vi "Z900_navX_SERIAL_DecodePacket.vi"(8 "error in (no error)":errorcluster, 10 "Data":u8[](array[numeric]), 11 "Packet":string) -> (0 "error out":errorcluster, 2 "Data":u8[](array[numeric]), 3 "Packet":string)   [LabVIEW 2015, in "navX Library v2.lvlib"]
uses:
  navX Library v2.lvlib
  TypeDefs/Z900_navX_DeviceRegisters.ctl
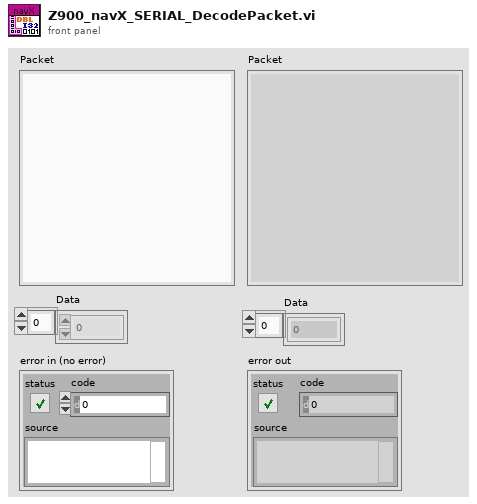
[diagram p1: front panel]
types:
  T1 = typedef "navX Library v2.lvlib/Z900_navX_DeviceRegisters.ctl" = u8
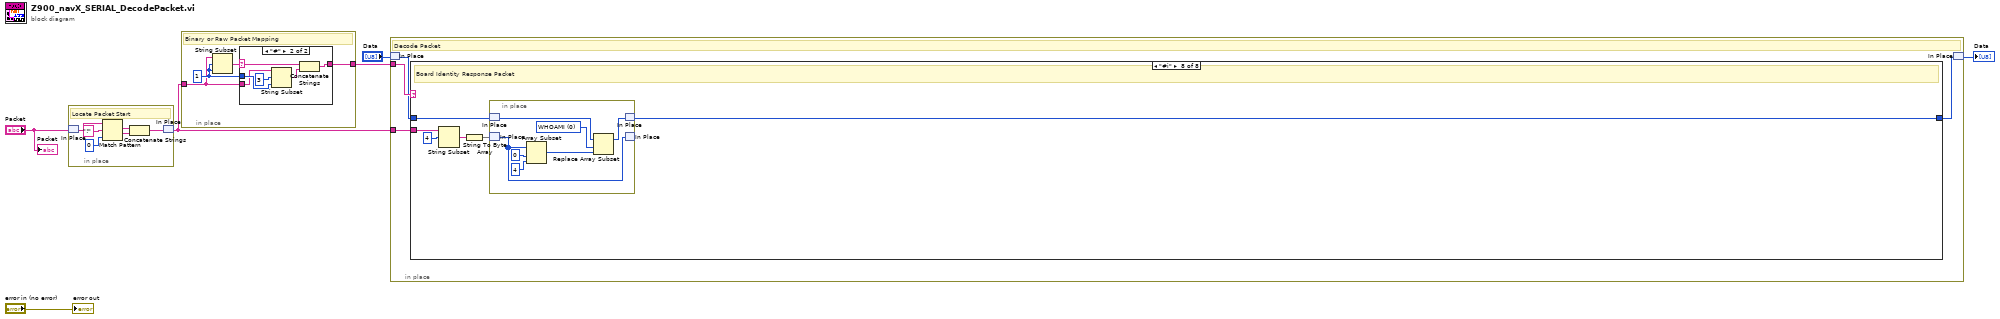
[diagram p0: block diagram]
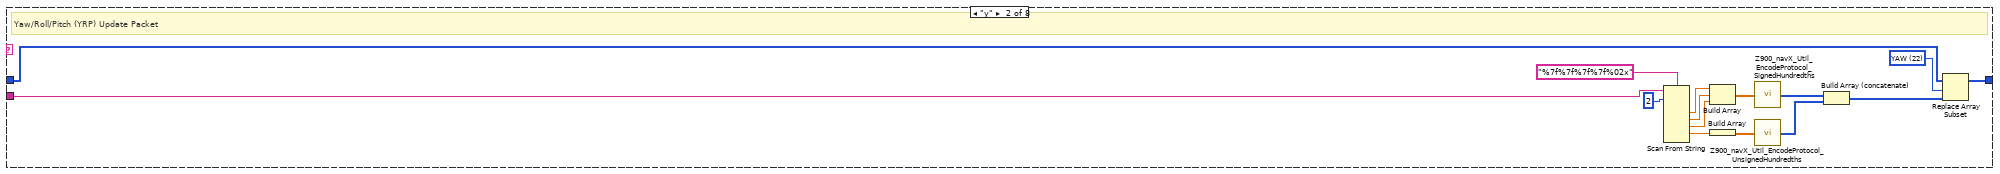
[diagram p3: hidden frame]
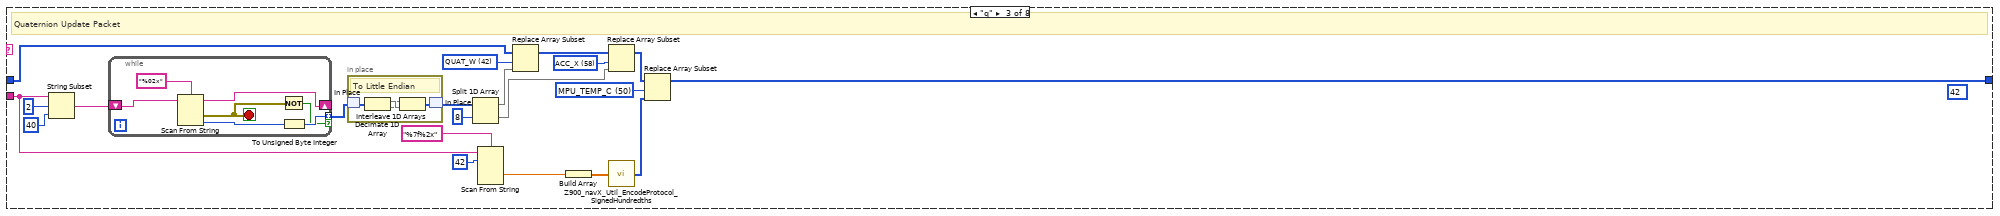
[diagram p4: hidden frame]
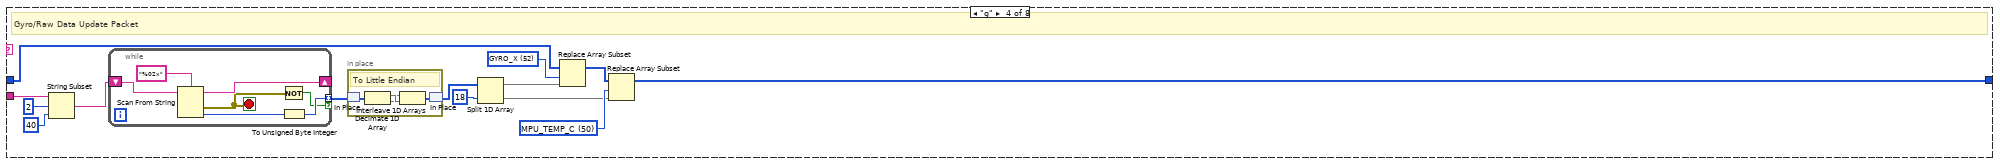
[diagram p5: hidden frame]
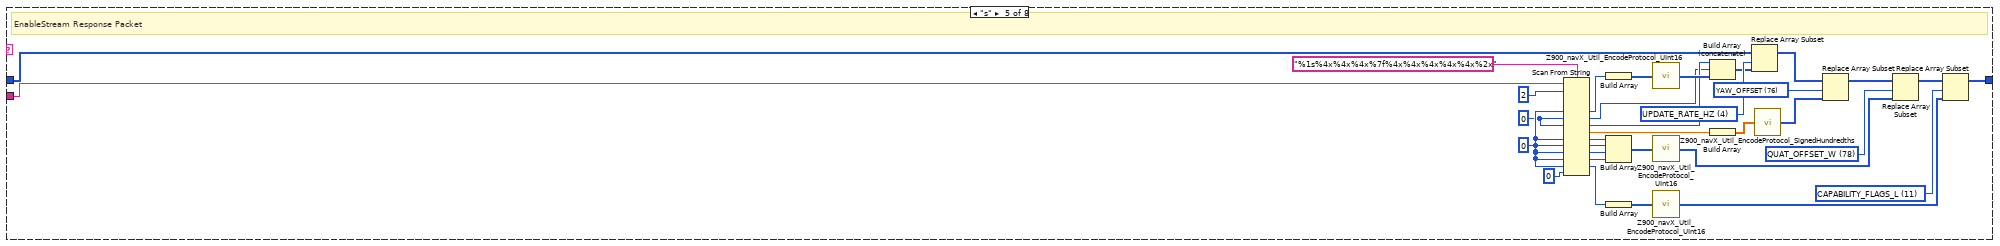
[diagram p6: hidden frame]
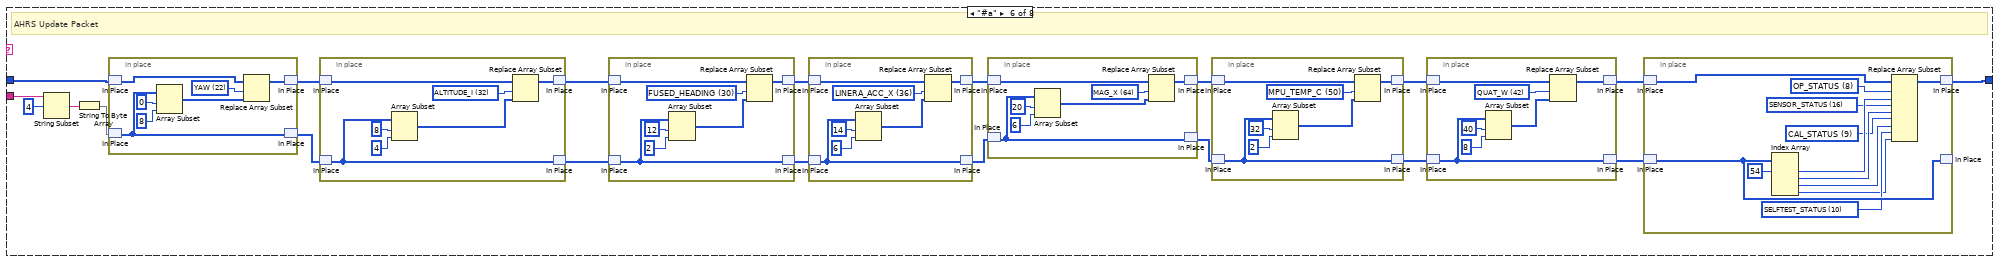
[diagram p7: hidden frame]
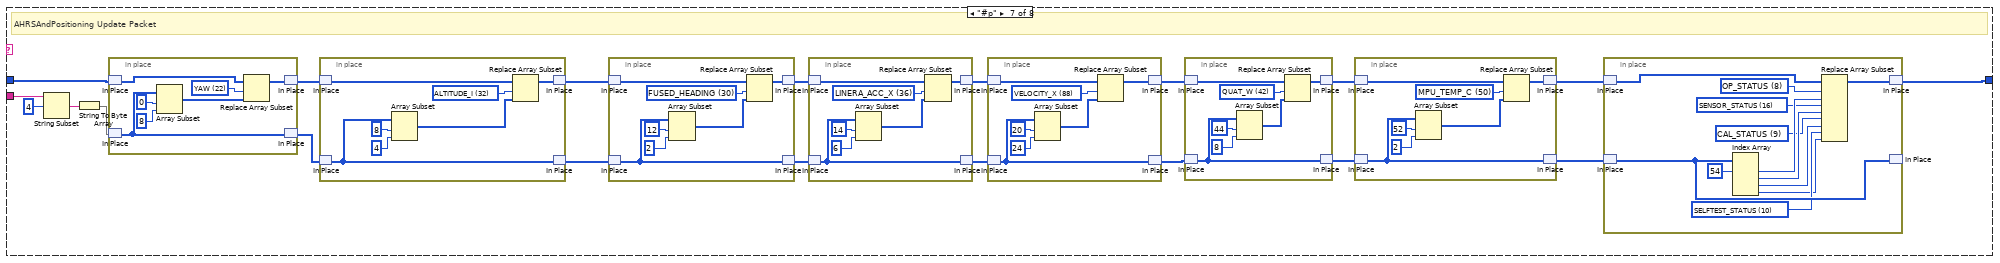
[diagram p8: hidden frame]
diagram:
  n1 = in-place {
    # "Locate Packet Start"
    n2 = in-place-match #1("Packet") -> (w8:string)
    n3 = Match Pattern(string=w8, regular expression="!" ("Packet Start Char"), offset (0)=0 ("offset past match")) -> (match substring=w11:string, after substring=w10:string)  [unwired: 2 out]
    n4 = Concatenate Strings(w11, w10) -> (w7:string)
    n5 = in-place-match #1(w7) -> (w2:string)
  }
  n6 = in-place {
    in-place-border: w2 -> [w14]
    in-place-border: [w16] -> w3
    w15 = 1 ("length (rest)")
    # "Binary or Raw Packet Mapping"
    n7 = String Subset(string=w14, offset (0)=w15, length (rest)=w15) -> (substring=w13:string)
    n8 = case shown="\"#\"" w13 {
      selector: w13 -> [w17 w18]
      tunnel: [w17 w19] -> w16
      tunnel: w15 -> [_ w22]
      tunnel: w14 -> [_ w21]
      frame Default {
      }
      frame "#" {
        n9 = String Subset(string=w21, offset (0)=3, length (rest)=w22) -> (substring=w20:string)
        n10 = Concatenate Strings(w18, w20) -> (w19:string)
      }
    }
  }
  n11 = in-place {
    in-place-border: w3 -> [w27]
    in-place-border: w2 -> [w25]
    # "Decode Packet"
    n12 = in-place-match #2("Data") -> (w26:u8[])
    n13 = case shown="\"#i\"" w27 {
      tunnel: w26 -> [w28 w34 w48 w85 w122 w150 w230 w297]
      tunnel: [w28 w29 w54 w78 w111 w134 w215 w296] -> w24
      tunnel: w25 -> [_ w41 w59 w87 w128 w153 w231 w299]
      frame Default {
        # "We should not care about decoding this packet type."
        # "Unknown Packet"
      }
      frame "y" {
        w30 = T1 22 items=["WHOAMI"=0, "HW_REV"=1, "FW_VER_MAJOR"=2, "FW_VER_MINOR"=3, "UPDATE_RATE_HZ"=4, "ACCEL_FSR_G"=5, "GYRO_FSR_DPS"=6, "OP_STATUS"=8, "CAL_STATUS"=9, "SELFTEST_STATUS"=10, "CAPABILITY_FLAGS_L"=11, "CAPABILITY_FLAGS_H"=12, "SENSOR_STATUS"=16, "TIMESTAMP"=18, "YAW"=22, "ROLL"=24, "PITCH"=26, "HEADING"=28, "FUSED_HEADING"=30, "ALTITUDE_I"=32, "ALTITUDE_D"=34, "LINERA_ACC_X"=36, "LINERA_ACC_Y"=38, "LINERA_ACC_Z"=40, "QUAT_W"=42, "QUAT_X"=44, "QUAT_Y"=46, "QUAT_Z"=48, "MPU_TEMP_C"=50, "GYRO_X"=52, "GYRO_Y"=54, "GYRO_Z"=56, "ACC_X"=58, "ACC_Y"=60, "ACC_Z"=62, "MAG_X"=64, "MAG_Y"=66, "MAG_Z"=68, "PRESSURE_I"=70, "PRESSURE_D"=72, "PRESSURE_TEMP"=74, "YAW_OFFSET"=76, "QUAT_OFFSET_W"=78, "QUAT_OFFSET_X"=80, "QUAT_OFFSET_Y"=82, "QUAT_OFFSET_Z"=84, "INTEGRATION_CONTROL"=86, "VELOCITY_X"=88, "VELOCITY_Y"=92, "VELOCITY_Z"=96, "DISPLACMENT_X"=100, "DISPLACMENT_Y"=104, "DISPLACEMENT_Z"=108] ("Device Register")
        # "Yaw/Roll/Pitch (YRP) Update Packet"
        n14 = Scan From String(format string="%7f%7f%7f%7f%02x", input string=w41, initial scan location=2 ("offset (0)")) -> (output 1=w40:dbl, output 2=w39:dbl, output 3=w38:dbl, output 4=w36:dbl)  [unwired: 7 in, 3 out]
        n15 = Build Array(w40, w39, w38) -> (w37:dbl[])
        n16 = Build Array(w36) -> (w35:dbl[])
        n17 = call "Z900_navX_Util_EncodeProtocol_SignedHundredths.vi"("Signed Hundredths (0.00)"=w37) -> ("Little Endian"=w33:u8[])
        n18 = call "Z900_navX_Util_EncodeProtocol_UnsignedHundredths.vi"("Unsigned Hundredths (0.00)"=w35) -> ("Little Endian"=w32:u8[])
        n19 = Build Array (concatenate)(w33, w32) -> (w31:u8[])
        n20 = Replace Array Subset(array=w34, new element=w31, index=w30) -> (w29:u8[])
      }
      frame "q" {
        w44 = T1 42 items=["WHOAMI"=0, "HW_REV"=1, "FW_VER_MAJOR"=2, "FW_VER_MINOR"=3, "UPDATE_RATE_HZ"=4, "ACCEL_FSR_G"=5, "GYRO_FSR_DPS"=6, "OP_STATUS"=8, "CAL_STATUS"=9, "SELFTEST_STATUS"=10, "CAPABILITY_FLAGS_L"=11, "CAPABILITY_FLAGS_H"=12, "SENSOR_STATUS"=16, "TIMESTAMP"=18, "YAW"=22, "ROLL"=24, "PITCH"=26, "HEADING"=28, "FUSED_HEADING"=30, "ALTITUDE_I"=32, "ALTITUDE_D"=34, "LINERA_ACC_X"=36, "LINERA_ACC_Y"=38, "LINERA_ACC_Z"=40, "QUAT_W"=42, "QUAT_X"=44, "QUAT_Y"=46, "QUAT_Z"=48, "MPU_TEMP_C"=50, "GYRO_X"=52, "GYRO_Y"=54, "GYRO_Z"=56, "ACC_X"=58, "ACC_Y"=60, "ACC_Z"=62, "MAG_X"=64, "MAG_Y"=66, "MAG_Z"=68, "PRESSURE_I"=70, "PRESSURE_D"=72, "PRESSURE_TEMP"=74, "YAW_OFFSET"=76, "QUAT_OFFSET_W"=78, "QUAT_OFFSET_X"=80, "QUAT_OFFSET_Y"=82, "QUAT_OFFSET_Z"=84, "INTEGRATION_CONTROL"=86, "VELOCITY_X"=88, "VELOCITY_Y"=92, "VELOCITY_Z"=96, "DISPLACMENT_X"=100, "DISPLACMENT_Y"=104, "DISPLACEMENT_Z"=108] ("Device Register")
        w51 = T1 58 items=["WHOAMI"=0, "HW_REV"=1, "FW_VER_MAJOR"=2, "FW_VER_MINOR"=3, "UPDATE_RATE_HZ"=4, "ACCEL_FSR_G"=5, "GYRO_FSR_DPS"=6, "OP_STATUS"=8, "CAL_STATUS"=9, "SELFTEST_STATUS"=10, "CAPABILITY_FLAGS_L"=11, "CAPABILITY_FLAGS_H"=12, "SENSOR_STATUS"=16, "TIMESTAMP"=18, "YAW"=22, "ROLL"=24, "PITCH"=26, "HEADING"=28, "FUSED_HEADING"=30, "ALTITUDE_I"=32, "ALTITUDE_D"=34, "LINERA_ACC_X"=36, "LINERA_ACC_Y"=38, "LINERA_ACC_Z"=40, "QUAT_W"=42, "QUAT_X"=44, "QUAT_Y"=46, "QUAT_Z"=48, "MPU_TEMP_C"=50, "GYRO_X"=52, "GYRO_Y"=54, "GYRO_Z"=56, "ACC_X"=58, "ACC_Y"=60, "ACC_Z"=62, "MAG_X"=64, "MAG_Y"=66, "MAG_Z"=68, "PRESSURE_I"=70, "PRESSURE_D"=72, "PRESSURE_TEMP"=74, "YAW_OFFSET"=76, "QUAT_OFFSET_W"=78, "QUAT_OFFSET_X"=80, "QUAT_OFFSET_Y"=82, "QUAT_OFFSET_Z"=84, "INTEGRATION_CONTROL"=86, "VELOCITY_X"=88, "VELOCITY_Y"=92, "VELOCITY_Z"=96, "DISPLACMENT_X"=100, "DISPLACMENT_Y"=104, "DISPLACEMENT_Z"=108] ("Device Register")
        (unwired) T1 42 items=["WHOAMI"=0, "HW_REV"=1, "FW_VER_MAJOR"=2, "FW_VER_MINOR"=3, "UPDATE_RATE_HZ"=4, "ACCEL_FSR_G"=5, "GYRO_FSR_DPS"=6, "OP_STATUS"=8, "CAL_STATUS"=9, "SELFTEST_STATUS"=10, "CAPABILITY_FLAGS_L"=11, "CAPABILITY_FLAGS_H"=12, "SENSOR_STATUS"=16, "TIMESTAMP"=18, "YAW"=22, "ROLL"=24, "PITCH"=26, "HEADING"=28, "FUSED_HEADING"=30, "ALTITUDE_I"=32, "ALTITUDE_D"=34, "LINERA_ACC_X"=36, "LINERA_ACC_Y"=38, "LINERA_ACC_Z"=40, ""=42, "QUAT_X"=44, "QUAT_Y"=46, "QUAT_Z"=48, "MPU_TEMP_C"=50, "GYRO_X"=52, "GYRO_Y"=54, "GYRO_Z"=56, "ACC_X"=58, "ACC_Y"=60, "ACC_Z"=62, "MAG_X"=64, "MAG_Y"=66, "MAG_Z"=68, "PRESSURE_I"=70, "PRESSURE_D"=72, "PRESSURE_TEMP"=74, "YAW_OFFSET"=76, "QUAT_OFFSET_W"=78, "QUAT_OFFSET_X"=80, "QUAT_OFFSET_Y"=82, "QUAT_OFFSET_Z"=84, "INTEGRATION_CONTROL"=86, "VELOCITY_X"=88, "VELOCITY_Y"=92, "VELOCITY_Z"=96, "DISPLACMENT_X"=100, "DISPLACMENT_Y"=104, "DISPLACEMENT_Z"=108] ("Device Register")
        w56 = T1 50 items=["WHOAMI"=0, "HW_REV"=1, "FW_VER_MAJOR"=2, "FW_VER_MINOR"=3, "UPDATE_RATE_HZ"=4, "ACCEL_FSR_G"=5, "GYRO_FSR_DPS"=6, "OP_STATUS"=8, "CAL_STATUS"=9, "SELFTEST_STATUS"=10, "CAPABILITY_FLAGS_L"=11, "CAPABILITY_FLAGS_H"=12, "SENSOR_STATUS"=16, "TIMESTAMP"=18, "YAW"=22, "ROLL"=24, "PITCH"=26, "HEADING"=28, "FUSED_HEADING"=30, "ALTITUDE_I"=32, "ALTITUDE_D"=34, "LINERA_ACC_X"=36, "LINERA_ACC_Y"=38, "LINERA_ACC_Z"=40, "QUAT_W"=42, "QUAT_X"=44, "QUAT_Y"=46, "QUAT_Z"=48, "MPU_TEMP_C"=50, "GYRO_X"=52, "GYRO_Y"=54, "GYRO_Z"=56, "ACC_X"=58, "ACC_Y"=60, "ACC_Z"=62, "MAG_X"=64, "MAG_Y"=66, "MAG_Z"=68, "PRESSURE_I"=70, "PRESSURE_D"=72, "PRESSURE_TEMP"=74, "YAW_OFFSET"=76, "QUAT_OFFSET_W"=78, "QUAT_OFFSET_X"=80, "QUAT_OFFSET_Y"=82, "QUAT_OFFSET_Z"=84, "INTEGRATION_CONTROL"=86, "VELOCITY_X"=88, "VELOCITY_Y"=92, "VELOCITY_Z"=96, "DISPLACMENT_X"=100, "DISPLACMENT_Y"=104, "DISPLACEMENT_Z"=108] ("Device Register")
        # "Quaternion Update Packet"
        n21 = String Subset(string=w59, offset (0)=2, length (rest)=40 ("length (rest)")) -> (substring=w61:string)
        n22 = while {
          shift-right: [w73] -> _
          shift-left: w61 -> [w74]
          tunnel: [w71] -> w50 mode=indexing if=w69
          stop <- w70 stop-if-true
          n23 = Scan From String(format string="%02x", input string=w74) -> (remaining string=w73:string, error out=w70:errorcluster, output 1=w72:u32)  [unwired: 3 in, 1 out]
          n24 = Not(x=w70) -> (.not. x?=w69:bool)
          n25 = To Unsigned Byte Integer(number=w72) -> (unsigned 8bit integer=w71:u8)
        }
        n26 = in-place {
          # "To Little Endian"
          n27 = in-place-match #3(w50) -> (w66:u8[])
          n28 = Decimate 1D Array(w66) -> (w68:u8[], w67:u8[])
          n29 = Interleave 1D Arrays(w67, w68) -> (w65:u8[])
          n30 = in-place-match #3(w65) -> (w49:u8[])
        }
        n31 = Split 1D Array(array=w49, index=8) -> (first subarray=w46:u8[], second subarray=w45:u8[])
        n32 = Scan From String(format string="%7f%2x", input string=w59, initial scan location=u32 42) -> (output 1=w57:dbl)  [unwired: 4 in, 3 out]
        n33 = Replace Array Subset(array=w48, new element=w46, index=w44) -> (w47:u8[])
        n34 = Build Array(w57) -> (w58:dbl[])
        n35 = Replace Array Subset(array=w47, new element=w45, index=w51) -> (w52:u8[])
        n36 = call "Z900_navX_Util_EncodeProtocol_SignedHundredths.vi"("Signed Hundredths (0.00)"=w58) -> ("Little Endian"=w55:u8[])
        n37 = Replace Array Subset(array=w52, new element=w55, index=w56) -> (w54:u8[])
      }
      frame "g" {
        w80 = T1 50 items=["WHOAMI"=0, "HW_REV"=1, "FW_VER_MAJOR"=2, "FW_VER_MINOR"=3, "UPDATE_RATE_HZ"=4, "ACCEL_FSR_G"=5, "GYRO_FSR_DPS"=6, "OP_STATUS"=8, "CAL_STATUS"=9, "SELFTEST_STATUS"=10, "CAPABILITY_FLAGS_L"=11, "CAPABILITY_FLAGS_H"=12, "SENSOR_STATUS"=16, "TIMESTAMP"=18, "YAW"=22, "ROLL"=24, "PITCH"=26, "HEADING"=28, "FUSED_HEADING"=30, "ALTITUDE_I"=32, "ALTITUDE_D"=34, "LINERA_ACC_X"=36, "LINERA_ACC_Y"=38, "LINERA_ACC_Z"=40, "QUAT_W"=42, "QUAT_X"=44, "QUAT_Y"=46, "QUAT_Z"=48, "MPU_TEMP_C"=50, "GYRO_X"=52, "GYRO_Y"=54, "GYRO_Z"=56, "ACC_X"=58, "ACC_Y"=60, "ACC_Z"=62, "MAG_X"=64, "MAG_Y"=66, "MAG_Z"=68, "PRESSURE_I"=70, "PRESSURE_D"=72, "PRESSURE_TEMP"=74, "YAW_OFFSET"=76, "QUAT_OFFSET_W"=78, "QUAT_OFFSET_X"=80, "QUAT_OFFSET_Y"=82, "QUAT_OFFSET_Z"=84, "INTEGRATION_CONTROL"=86, "VELOCITY_X"=88, "VELOCITY_Y"=92, "VELOCITY_Z"=96, "DISPLACMENT_X"=100, "DISPLACMENT_Y"=104, "DISPLACEMENT_Z"=108] ("Device Register")
        w84 = T1 52 items=["WHOAMI"=0, "HW_REV"=1, "FW_VER_MAJOR"=2, "FW_VER_MINOR"=3, "UPDATE_RATE_HZ"=4, "ACCEL_FSR_G"=5, "GYRO_FSR_DPS"=6, "OP_STATUS"=8, "CAL_STATUS"=9, "SELFTEST_STATUS"=10, "CAPABILITY_FLAGS_L"=11, "CAPABILITY_FLAGS_H"=12, "SENSOR_STATUS"=16, "TIMESTAMP"=18, "YAW"=22, "ROLL"=24, "PITCH"=26, "HEADING"=28, "FUSED_HEADING"=30, "ALTITUDE_I"=32, "ALTITUDE_D"=34, "LINERA_ACC_X"=36, "LINERA_ACC_Y"=38, "LINERA_ACC_Z"=40, "QUAT_W"=42, "QUAT_X"=44, "QUAT_Y"=46, "QUAT_Z"=48, "MPU_TEMP_C"=50, "GYRO_X"=52, "GYRO_Y"=54, "GYRO_Z"=56, "ACC_X"=58, "ACC_Y"=60, "ACC_Z"=62, "MAG_X"=64, "MAG_Y"=66, "MAG_Z"=68, "PRESSURE_I"=70, "PRESSURE_D"=72, "PRESSURE_TEMP"=74, "YAW_OFFSET"=76, "QUAT_OFFSET_W"=78, "QUAT_OFFSET_X"=80, "QUAT_OFFSET_Y"=82, "QUAT_OFFSET_Z"=84, "INTEGRATION_CONTROL"=86, "VELOCITY_X"=88, "VELOCITY_Y"=92, "VELOCITY_Z"=96, "DISPLACMENT_X"=100, "DISPLACMENT_Y"=104, "DISPLACEMENT_Z"=108] ("Device Register")
        # "Gyro/Raw Data Update Packet"
        n38 = String Subset(string=w87, offset (0)=2, length (rest)=40 ("length (rest)")) -> (substring=w86:string)
        n39 = while {
          shift-right: [w98] -> _
          shift-left: w86 -> [w99]
          tunnel: [w96] -> w77 mode=indexing if=w94
          stop <- w95 stop-if-true
          n40 = Scan From String(format string="%02x", input string=w99) -> (remaining string=w98:string, error out=w95:errorcluster, output 1=w97:u32)  [unwired: 3 in, 1 out]
          n41 = Not(x=w95) -> (.not. x?=w94:bool)
          n42 = To Unsigned Byte Integer(number=w97) -> (unsigned 8bit integer=w96:u8)
        }
        n43 = in-place {
          # "To Little Endian"
          n44 = in-place-match #4(w77) -> (w91:u8[])
          n45 = Decimate 1D Array(w91) -> (w93:u8[], w92:u8[])
          n46 = Interleave 1D Arrays(w92, w93) -> (w90:u8[])
          n47 = in-place-match #4(w90) -> (w76:u8[])
        }
        n48 = Split 1D Array(array=w76, index=18) -> (first subarray=w83:u8[], second subarray=w79:u8[])
        n49 = Replace Array Subset(array=w85, new element=w83, index=w84) -> (w81:u8[])
        n50 = Replace Array Subset(array=w81, new element=w79, index=w80) -> (w78:u8[])
      }
      frame "s" {
        w104 = u8 0 ("default value 2")
        w113 = T1 11 items=["WHOAMI"=0, "HW_REV"=1, "FW_VER_MAJOR"=2, "FW_VER_MINOR"=3, "UPDATE_RATE_HZ"=4, "ACCEL_FSR_G"=5, "GYRO_FSR_DPS"=6, "OP_STATUS"=8, "CAL_STATUS"=9, "SELFTEST_STATUS"=10, "CAPABILITY_FLAGS_L"=11, "CAPABILITY_FLAGS_H"=12, "SENSOR_STATUS"=16, "TIMESTAMP"=18, "YAW"=22, "ROLL"=24, "PITCH"=26, "HEADING"=28, "FUSED_HEADING"=30, "ALTITUDE_I"=32, "ALTITUDE_D"=34, "LINERA_ACC_X"=36, "LINERA_ACC_Y"=38, "LINERA_ACC_Z"=40, "QUAT_W"=42, "QUAT_X"=44, "QUAT_Y"=46, "QUAT_Z"=48, "MPU_TEMP_C"=50, "GYRO_X"=52, "GYRO_Y"=54, "GYRO_Z"=56, "ACC_X"=58, "ACC_Y"=60, "ACC_Z"=62, "MAG_X"=64, "MAG_Y"=66, "MAG_Z"=68, "PRESSURE_I"=70, "PRESSURE_D"=72, "PRESSURE_TEMP"=74, "YAW_OFFSET"=76, "QUAT_OFFSET_W"=78, "QUAT_OFFSET_X"=80, "QUAT_OFFSET_Y"=82, "QUAT_OFFSET_Z"=84, "INTEGRATION_CONTROL"=86, "VELOCITY_X"=88, "VELOCITY_Y"=92, "VELOCITY_Z"=96, "DISPLACMENT_X"=100, "DISPLACMENT_Y"=104, "DISPLACEMENT_Z"=108] ("Device Register")
        w116 = T1 78 items=["WHOAMI"=0, "HW_REV"=1, "FW_VER_MAJOR"=2, "FW_VER_MINOR"=3, "UPDATE_RATE_HZ"=4, "ACCEL_FSR_G"=5, "GYRO_FSR_DPS"=6, "OP_STATUS"=8, "CAL_STATUS"=9, "SELFTEST_STATUS"=10, "CAPABILITY_FLAGS_L"=11, "CAPABILITY_FLAGS_H"=12, "SENSOR_STATUS"=16, "TIMESTAMP"=18, "YAW"=22, "ROLL"=24, "PITCH"=26, "HEADING"=28, "FUSED_HEADING"=30, "ALTITUDE_I"=32, "ALTITUDE_D"=34, "LINERA_ACC_X"=36, "LINERA_ACC_Y"=38, "LINERA_ACC_Z"=40, "QUAT_W"=42, "QUAT_X"=44, "QUAT_Y"=46, "QUAT_Z"=48, "MPU_TEMP_C"=50, "GYRO_X"=52, "GYRO_Y"=54, "GYRO_Z"=56, "ACC_X"=58, "ACC_Y"=60, "ACC_Z"=62, "MAG_X"=64, "MAG_Y"=66, "MAG_Z"=68, "PRESSURE_I"=70, "PRESSURE_D"=72, "PRESSURE_TEMP"=74, "YAW_OFFSET"=76, "QUAT_OFFSET_W"=78, "QUAT_OFFSET_X"=80, "QUAT_OFFSET_Y"=82, "QUAT_OFFSET_Z"=84, "INTEGRATION_CONTROL"=86, "VELOCITY_X"=88, "VELOCITY_Y"=92, "VELOCITY_Z"=96, "DISPLACMENT_X"=100, "DISPLACMENT_Y"=104, "DISPLACEMENT_Z"=108] ("Device Register")
        w119 = T1 76 items=["WHOAMI"=0, "HW_REV"=1, "FW_VER_MAJOR"=2, "FW_VER_MINOR"=3, "UPDATE_RATE_HZ"=4, "ACCEL_FSR_G"=5, "GYRO_FSR_DPS"=6, "OP_STATUS"=8, "CAL_STATUS"=9, "SELFTEST_STATUS"=10, "CAPABILITY_FLAGS_L"=11, "CAPABILITY_FLAGS_H"=12, "SENSOR_STATUS"=16, "TIMESTAMP"=18, "YAW"=22, "ROLL"=24, "PITCH"=26, "HEADING"=28, "FUSED_HEADING"=30, "ALTITUDE_I"=32, "ALTITUDE_D"=34, "LINERA_ACC_X"=36, "LINERA_ACC_Y"=38, "LINERA_ACC_Z"=40, "QUAT_W"=42, "QUAT_X"=44, "QUAT_Y"=46, "QUAT_Z"=48, "MPU_TEMP_C"=50, "GYRO_X"=52, "GYRO_Y"=54, "GYRO_Z"=56, "ACC_X"=58, "ACC_Y"=60, "ACC_Z"=62, "MAG_X"=64, "MAG_Y"=66, "MAG_Z"=68, "PRESSURE_I"=70, "PRESSURE_D"=72, "PRESSURE_TEMP"=74, "YAW_OFFSET"=76, "QUAT_OFFSET_W"=78, "QUAT_OFFSET_X"=80, "QUAT_OFFSET_Y"=82, "QUAT_OFFSET_Z"=84, "INTEGRATION_CONTROL"=86, "VELOCITY_X"=88, "VELOCITY_Y"=92, "VELOCITY_Z"=96, "DISPLACMENT_X"=100, "DISPLACMENT_Y"=104, "DISPLACEMENT_Z"=108] ("Device Register")
        w121 = T1 4 items=["WHOAMI"=0, "HW_REV"=1, "FW_VER_MAJOR"=2, "FW_VER_MINOR"=3, "UPDATE_RATE_HZ"=4, "ACCEL_FSR_G"=5, "GYRO_FSR_DPS"=6, "OP_STATUS"=8, "CAL_STATUS"=9, "SELFTEST_STATUS"=10, "CAPABILITY_FLAGS_L"=11, "CAPABILITY_FLAGS_H"=12, "SENSOR_STATUS"=16, "TIMESTAMP"=18, "YAW"=22, "ROLL"=24, "PITCH"=26, "HEADING"=28, "FUSED_HEADING"=30, "ALTITUDE_I"=32, "ALTITUDE_D"=34, "LINERA_ACC_X"=36, "LINERA_ACC_Y"=38, "LINERA_ACC_Z"=40, "QUAT_W"=42, "QUAT_X"=44, "QUAT_Y"=46, "QUAT_Z"=48, "MPU_TEMP_C"=50, "GYRO_X"=52, "GYRO_Y"=54, "GYRO_Z"=56, "ACC_X"=58, "ACC_Y"=60, "ACC_Z"=62, "MAG_X"=64, "MAG_Y"=66, "MAG_Z"=68, "PRESSURE_I"=70, "PRESSURE_D"=72, "PRESSURE_TEMP"=74, "YAW_OFFSET"=76, "QUAT_OFFSET_W"=78, "QUAT_OFFSET_X"=80, "QUAT_OFFSET_Y"=82, "QUAT_OFFSET_Z"=84, "INTEGRATION_CONTROL"=86, "VELOCITY_X"=88, "VELOCITY_Y"=92, "VELOCITY_Z"=96, "DISPLACMENT_X"=100, "DISPLACMENT_Y"=104, "DISPLACEMENT_Z"=108] ("Device Register")
        w105 = u16 0
        # "EnableStream Response Packet"
        n51 = Scan From String(format string="%1s%4x%4x%4x%7f%4x%4x%4x%4x%4x%2x", input string=w128, initial scan location=u32 2, default 2=w105, default 3=w104, default 4=w104, default 6=w105, default 7=w105, default 8=w105, default 9=w105, default 10=w105, default 11=u8 0) -> (output 2=w106:u16, output 3=w101:u8, output 4=w102:u8, output 5=w130:dbl, output 6=w127:u16, output 7=w126:u16, output 8=w125:u16, output 9=w124:u16, output 10=w110:u16)  [unwired: 5 in, 3 out]
        n52 = Build Array(w106) -> (w103:u16[])
        n53 = Build Array(w127, w126, w125, w124) -> (w123:u16[])
        n54 = Build Array(w110) -> (w109:u16[])
        n55 = call "Z900_navX_Util_EncodeProtocol_UInt16.vi"("UInt16"=w103) -> ("Little Endian"=w108:u8[])
        n56 = call "Z900_navX_Util_EncodeProtocol_UInt16.vi"("UInt16"=w123) -> ("Little Endian"=w115:u8[])
        n57 = call "Z900_navX_Util_EncodeProtocol_UInt16.vi"("UInt16"=w109) -> ("Little Endian"=w112:u8[])
        n58 = Build Array (concatenate)(w102, w101, w108) -> (w107:u8[])
        n59 = Build Array(w130) -> (w129:dbl[])
        n60 = Replace Array Subset(array=w122, new element=w107, index=w121) -> (w120:u8[])
        n61 = call "Z900_navX_Util_EncodeProtocol_SignedHundredths.vi"("Signed Hundredths (0.00)"=w129) -> ("Little Endian"=w118:u8[])
        n62 = Replace Array Subset(array=w120, new element=w118, index=w119) -> (w117:u8[])
        n63 = Replace Array Subset(array=w117, new element=w115, index=w116) -> (w114:u8[])
        n64 = Replace Array Subset(array=w114, new element=w112, index=w113) -> (w111:u8[])
      }
      frame "#a" {
        # "AHRS Update Packet"
        n65 = String Subset(string=w153, offset (0)=4) -> (substring=w151:string)  [unwired: 1 in]
        n66 = String To Byte Array(string=w151) -> (unsigned byte array=w148:u8[])
        n67 = in-place {
          w211 = T1 22 items=["WHOAMI"=0, "HW_REV"=1, "FW_VER_MAJOR"=2, "FW_VER_MINOR"=3, "UPDATE_RATE_HZ"=4, "ACCEL_FSR_G"=5, "GYRO_FSR_DPS"=6, "OP_STATUS"=8, "CAL_STATUS"=9, "SELFTEST_STATUS"=10, "CAPABILITY_FLAGS_L"=11, "CAPABILITY_FLAGS_H"=12, "SENSOR_STATUS"=16, "TIMESTAMP"=18, "YAW"=22, "ROLL"=24, "PITCH"=26, "HEADING"=28, "FUSED_HEADING"=30, "ALTITUDE_I"=32, "ALTITUDE_D"=34, "LINERA_ACC_X"=36, "LINERA_ACC_Y"=38, "LINERA_ACC_Z"=40, "QUAT_W"=42, "QUAT_X"=44, "QUAT_Y"=46, "QUAT_Z"=48, "MPU_TEMP_C"=50, "GYRO_X"=52, "GYRO_Y"=54, "GYRO_Z"=56, "ACC_X"=58, "ACC_Y"=60, "ACC_Z"=62, "MAG_X"=64, "MAG_Y"=66, "MAG_Z"=68, "PRESSURE_I"=70, "PRESSURE_D"=72, "PRESSURE_TEMP"=74, "YAW_OFFSET"=76, "QUAT_OFFSET_W"=78, "QUAT_OFFSET_X"=80, "QUAT_OFFSET_Y"=82, "QUAT_OFFSET_Z"=84, "INTEGRATION_CONTROL"=86, "VELOCITY_X"=88, "VELOCITY_Y"=92, "VELOCITY_Z"=96, "DISPLACMENT_X"=100, "DISPLACMENT_Y"=104, "DISPLACEMENT_Z"=108] ("Device Register")
          n68 = in-place-match #5(w150) -> (w210:u8[])
          n69 = in-place-match #6(w148) -> (w208:u8[])
          n70 = Array Subset(array=w208, index=0, length=8) -> (w212:u8[])
          n71 = Replace Array Subset(array=w210, new element=w212, index=w211) -> (w209:u8[])
          n72 = in-place-match #5(w209) -> (w149:u8[])
          n73 = in-place-match #6(w208) -> (w147:u8[])
        }
        n74 = in-place {
          w205 = T1 32 items=["WHOAMI"=0, "HW_REV"=1, "FW_VER_MAJOR"=2, "FW_VER_MINOR"=3, "UPDATE_RATE_HZ"=4, "ACCEL_FSR_G"=5, "GYRO_FSR_DPS"=6, "OP_STATUS"=8, "CAL_STATUS"=9, "SELFTEST_STATUS"=10, "CAPABILITY_FLAGS_L"=11, "CAPABILITY_FLAGS_H"=12, "SENSOR_STATUS"=16, "TIMESTAMP"=18, "YAW"=22, "ROLL"=24, "PITCH"=26, "HEADING"=28, "FUSED_HEADING"=30, "ALTITUDE_I"=32, "ALTITUDE_D"=34, "LINERA_ACC_X"=36, "LINERA_ACC_Y"=38, "LINERA_ACC_Z"=40, "QUAT_W"=42, "QUAT_X"=44, "QUAT_Y"=46, "QUAT_Z"=48, "MPU_TEMP_C"=50, "GYRO_X"=52, "GYRO_Y"=54, "GYRO_Z"=56, "ACC_X"=58, "ACC_Y"=60, "ACC_Z"=62, "MAG_X"=64, "MAG_Y"=66, "MAG_Z"=68, "PRESSURE_I"=70, "PRESSURE_D"=72, "PRESSURE_TEMP"=74, "YAW_OFFSET"=76, "QUAT_OFFSET_W"=78, "QUAT_OFFSET_X"=80, "QUAT_OFFSET_Y"=82, "QUAT_OFFSET_Z"=84, "INTEGRATION_CONTROL"=86, "VELOCITY_X"=88, "VELOCITY_Y"=92, "VELOCITY_Z"=96, "DISPLACMENT_X"=100, "DISPLACMENT_Y"=104, "DISPLACEMENT_Z"=108] ("Device Register")
          n75 = in-place-match #7(w149) -> (w204:u8[])
          n76 = in-place-match #8(w147) -> (w201:u8[])
          n77 = Array Subset(array=w201, index=8, length=4) -> (w202:u8[])
          n78 = Replace Array Subset(array=w204, new element=w202, index=w205) -> (w203:u8[])
          n79 = in-place-match #7(w203) -> (w146:u8[])
          n80 = in-place-match #8(w201) -> (w145:u8[])
        }
        n81 = in-place {
          w198 = T1 30 items=["WHOAMI"=0, "HW_REV"=1, "FW_VER_MAJOR"=2, "FW_VER_MINOR"=3, "UPDATE_RATE_HZ"=4, "ACCEL_FSR_G"=5, "GYRO_FSR_DPS"=6, "OP_STATUS"=8, "CAL_STATUS"=9, "SELFTEST_STATUS"=10, "CAPABILITY_FLAGS_L"=11, "CAPABILITY_FLAGS_H"=12, "SENSOR_STATUS"=16, "TIMESTAMP"=18, "YAW"=22, "ROLL"=24, "PITCH"=26, "HEADING"=28, "FUSED_HEADING"=30, "ALTITUDE_I"=32, "ALTITUDE_D"=34, "LINERA_ACC_X"=36, "LINERA_ACC_Y"=38, "LINERA_ACC_Z"=40, "QUAT_W"=42, "QUAT_X"=44, "QUAT_Y"=46, "QUAT_Z"=48, "MPU_TEMP_C"=50, "GYRO_X"=52, "GYRO_Y"=54, "GYRO_Z"=56, "ACC_X"=58, "ACC_Y"=60, "ACC_Z"=62, "MAG_X"=64, "MAG_Y"=66, "MAG_Z"=68, "PRESSURE_I"=70, "PRESSURE_D"=72, "PRESSURE_TEMP"=74, "YAW_OFFSET"=76, "QUAT_OFFSET_W"=78, "QUAT_OFFSET_X"=80, "QUAT_OFFSET_Y"=82, "QUAT_OFFSET_Z"=84, "INTEGRATION_CONTROL"=86, "VELOCITY_X"=88, "VELOCITY_Y"=92, "VELOCITY_Z"=96, "DISPLACMENT_X"=100, "DISPLACMENT_Y"=104, "DISPLACEMENT_Z"=108] ("Device Register")
          n82 = in-place-match #9(w146) -> (w197:u8[])
          n83 = in-place-match #10(w145) -> (w194:u8[])
          n84 = Array Subset(array=w194, index=12, length=2) -> (w195:u8[])
          n85 = Replace Array Subset(array=w197, new element=w195, index=w198) -> (w196:u8[])
          n86 = in-place-match #9(w196) -> (w144:u8[])
          n87 = in-place-match #10(w194) -> (w143:u8[])
        }
        n88 = in-place {
          w191 = T1 36 items=["WHOAMI"=0, "HW_REV"=1, "FW_VER_MAJOR"=2, "FW_VER_MINOR"=3, "UPDATE_RATE_HZ"=4, "ACCEL_FSR_G"=5, "GYRO_FSR_DPS"=6, "OP_STATUS"=8, "CAL_STATUS"=9, "SELFTEST_STATUS"=10, "CAPABILITY_FLAGS_L"=11, "CAPABILITY_FLAGS_H"=12, "SENSOR_STATUS"=16, "TIMESTAMP"=18, "YAW"=22, "ROLL"=24, "PITCH"=26, "HEADING"=28, "FUSED_HEADING"=30, "ALTITUDE_I"=32, "ALTITUDE_D"=34, "LINERA_ACC_X"=36, "LINERA_ACC_Y"=38, "LINERA_ACC_Z"=40, "QUAT_W"=42, "QUAT_X"=44, "QUAT_Y"=46, "QUAT_Z"=48, "MPU_TEMP_C"=50, "GYRO_X"=52, "GYRO_Y"=54, "GYRO_Z"=56, "ACC_X"=58, "ACC_Y"=60, "ACC_Z"=62, "MAG_X"=64, "MAG_Y"=66, "MAG_Z"=68, "PRESSURE_I"=70, "PRESSURE_D"=72, "PRESSURE_TEMP"=74, "YAW_OFFSET"=76, "QUAT_OFFSET_W"=78, "QUAT_OFFSET_X"=80, "QUAT_OFFSET_Y"=82, "QUAT_OFFSET_Z"=84, "INTEGRATION_CONTROL"=86, "VELOCITY_X"=88, "VELOCITY_Y"=92, "VELOCITY_Z"=96, "DISPLACMENT_X"=100, "DISPLACMENT_Y"=104, "DISPLACEMENT_Z"=108] ("Device Register")
          n89 = in-place-match #11(w144) -> (w190:u8[])
          n90 = in-place-match #12(w143) -> (w187:u8[])
          n91 = Array Subset(array=w187, index=14, length=6) -> (w188:u8[])
          n92 = Replace Array Subset(array=w190, new element=w188, index=w191) -> (w189:u8[])
          n93 = in-place-match #11(w189) -> (w142:u8[])
          n94 = in-place-match #12(w187) -> (w141:u8[])
        }
        n95 = in-place {
          w184 = T1 64 items=["WHOAMI"=0, "HW_REV"=1, "FW_VER_MAJOR"=2, "FW_VER_MINOR"=3, "UPDATE_RATE_HZ"=4, "ACCEL_FSR_G"=5, "GYRO_FSR_DPS"=6, "OP_STATUS"=8, "CAL_STATUS"=9, "SELFTEST_STATUS"=10, "CAPABILITY_FLAGS_L"=11, "CAPABILITY_FLAGS_H"=12, "SENSOR_STATUS"=16, "TIMESTAMP"=18, "YAW"=22, "ROLL"=24, "PITCH"=26, "HEADING"=28, "FUSED_HEADING"=30, "ALTITUDE_I"=32, "ALTITUDE_D"=34, "LINERA_ACC_X"=36, "LINERA_ACC_Y"=38, "LINERA_ACC_Z"=40, "QUAT_W"=42, "QUAT_X"=44, "QUAT_Y"=46, "QUAT_Z"=48, "MPU_TEMP_C"=50, "GYRO_X"=52, "GYRO_Y"=54, "GYRO_Z"=56, "ACC_X"=58, "ACC_Y"=60, "ACC_Z"=62, "MAG_X"=64, "MAG_Y"=66, "MAG_Z"=68, "PRESSURE_I"=70, "PRESSURE_D"=72, "PRESSURE_TEMP"=74, "YAW_OFFSET"=76, "QUAT_OFFSET_W"=78, "QUAT_OFFSET_X"=80, "QUAT_OFFSET_Y"=82, "QUAT_OFFSET_Z"=84, "INTEGRATION_CONTROL"=86, "VELOCITY_X"=88, "VELOCITY_Y"=92, "VELOCITY_Z"=96, "DISPLACMENT_X"=100, "DISPLACMENT_Y"=104, "DISPLACEMENT_Z"=108] ("Device Register")
          n96 = in-place-match #13(w142) -> (w183:u8[])
          n97 = in-place-match #14(w141) -> (w180:u8[])
          n98 = Array Subset(array=w180, index=20, length=6) -> (w181:u8[])
          n99 = Replace Array Subset(array=w183, new element=w181, index=w184) -> (w182:u8[])
          n100 = in-place-match #13(w182) -> (w140:u8[])
          n101 = in-place-match #14(w180) -> (w139:u8[])
        }
        n102 = in-place {
          w177 = T1 50 items=["WHOAMI"=0, "HW_REV"=1, "FW_VER_MAJOR"=2, "FW_VER_MINOR"=3, "UPDATE_RATE_HZ"=4, "ACCEL_FSR_G"=5, "GYRO_FSR_DPS"=6, "OP_STATUS"=8, "CAL_STATUS"=9, "SELFTEST_STATUS"=10, "CAPABILITY_FLAGS_L"=11, "CAPABILITY_FLAGS_H"=12, "SENSOR_STATUS"=16, "TIMESTAMP"=18, "YAW"=22, "ROLL"=24, "PITCH"=26, "HEADING"=28, "FUSED_HEADING"=30, "ALTITUDE_I"=32, "ALTITUDE_D"=34, "LINERA_ACC_X"=36, "LINERA_ACC_Y"=38, "LINERA_ACC_Z"=40, "QUAT_W"=42, "QUAT_X"=44, "QUAT_Y"=46, "QUAT_Z"=48, "MPU_TEMP_C"=50, "GYRO_X"=52, "GYRO_Y"=54, "GYRO_Z"=56, "ACC_X"=58, "ACC_Y"=60, "ACC_Z"=62, "MAG_X"=64, "MAG_Y"=66, "MAG_Z"=68, "PRESSURE_I"=70, "PRESSURE_D"=72, "PRESSURE_TEMP"=74, "YAW_OFFSET"=76, "QUAT_OFFSET_W"=78, "QUAT_OFFSET_X"=80, "QUAT_OFFSET_Y"=82, "QUAT_OFFSET_Z"=84, "INTEGRATION_CONTROL"=86, "VELOCITY_X"=88, "VELOCITY_Y"=92, "VELOCITY_Z"=96, "DISPLACMENT_X"=100, "DISPLACMENT_Y"=104, "DISPLACEMENT_Z"=108] ("Device Register")
          n103 = in-place-match #15(w140) -> (w176:u8[])
          n104 = in-place-match #16(w139) -> (w173:u8[])
          n105 = Array Subset(array=w173, index=32, length=2) -> (w174:u8[])
          n106 = Replace Array Subset(array=w176, new element=w174, index=w177) -> (w175:u8[])
          n107 = in-place-match #15(w175) -> (w137:u8[])
          n108 = in-place-match #16(w173) -> (w138:u8[])
        }
        n109 = in-place {
          w170 = T1 42 items=["WHOAMI"=0, "HW_REV"=1, "FW_VER_MAJOR"=2, "FW_VER_MINOR"=3, "UPDATE_RATE_HZ"=4, "ACCEL_FSR_G"=5, "GYRO_FSR_DPS"=6, "OP_STATUS"=8, "CAL_STATUS"=9, "SELFTEST_STATUS"=10, "CAPABILITY_FLAGS_L"=11, "CAPABILITY_FLAGS_H"=12, "SENSOR_STATUS"=16, "TIMESTAMP"=18, "YAW"=22, "ROLL"=24, "PITCH"=26, "HEADING"=28, "FUSED_HEADING"=30, "ALTITUDE_I"=32, "ALTITUDE_D"=34, "LINERA_ACC_X"=36, "LINERA_ACC_Y"=38, "LINERA_ACC_Z"=40, "QUAT_W"=42, "QUAT_X"=44, "QUAT_Y"=46, "QUAT_Z"=48, "MPU_TEMP_C"=50, "GYRO_X"=52, "GYRO_Y"=54, "GYRO_Z"=56, "ACC_X"=58, "ACC_Y"=60, "ACC_Z"=62, "MAG_X"=64, "MAG_Y"=66, "MAG_Z"=68, "PRESSURE_I"=70, "PRESSURE_D"=72, "PRESSURE_TEMP"=74, "YAW_OFFSET"=76, "QUAT_OFFSET_W"=78, "QUAT_OFFSET_X"=80, "QUAT_OFFSET_Y"=82, "QUAT_OFFSET_Z"=84, "INTEGRATION_CONTROL"=86, "VELOCITY_X"=88, "VELOCITY_Y"=92, "VELOCITY_Z"=96, "DISPLACMENT_X"=100, "DISPLACMENT_Y"=104, "DISPLACEMENT_Z"=108] ("Device Register")
          n110 = in-place-match #17(w137) -> (w169:u8[])
          n111 = in-place-match #18(w138) -> (w166:u8[])
          n112 = Array Subset(array=w166, index=40, length=8) -> (w167:u8[])
          n113 = Replace Array Subset(array=w169, new element=w167, index=w170) -> (w168:u8[])
          n114 = in-place-match #17(w168) -> (w136:u8[])
          n115 = in-place-match #18(w166) -> (w135:u8[])
        }
        n116 = in-place {
          w156 = T1 10 items=["WHOAMI"=0, "HW_REV"=1, "FW_VER_MAJOR"=2, "FW_VER_MINOR"=3, "UPDATE_RATE_HZ"=4, "ACCEL_FSR_G"=5, "GYRO_FSR_DPS"=6, "OP_STATUS"=8, "CAL_STATUS"=9, "SELFTEST_STATUS"=10, "CAPABILITY_FLAGS_L"=11, "CAPABILITY_FLAGS_H"=12, "SENSOR_STATUS"=16, "TIMESTAMP"=18, "YAW"=22, "ROLL"=24, "PITCH"=26, "HEADING"=28, "FUSED_HEADING"=30, "ALTITUDE_I"=32, "ALTITUDE_D"=34, "LINERA_ACC_X"=36, "LINERA_ACC_Y"=38, "LINERA_ACC_Z"=40, "QUAT_W"=42, "QUAT_X"=44, "QUAT_Y"=46, "QUAT_Z"=48, "MPU_TEMP_C"=50, "GYRO_X"=52, "GYRO_Y"=54, "GYRO_Z"=56, "ACC_X"=58, "ACC_Y"=60, "ACC_Z"=62, "MAG_X"=64, "MAG_Y"=66, "MAG_Z"=68, "PRESSURE_I"=70, "PRESSURE_D"=72, "PRESSURE_TEMP"=74, "YAW_OFFSET"=76, "QUAT_OFFSET_W"=78, "QUAT_OFFSET_X"=80, "QUAT_OFFSET_Y"=82, "QUAT_OFFSET_Z"=84, "INTEGRATION_CONTROL"=86, "VELOCITY_X"=88, "VELOCITY_Y"=92, "VELOCITY_Z"=96, "DISPLACMENT_X"=100, "DISPLACMENT_Y"=104, "DISPLACEMENT_Z"=108] ("Device Register")
          w157 = T1 9 items=["WHOAMI"=0, "HW_REV"=1, "FW_VER_MAJOR"=2, "FW_VER_MINOR"=3, "UPDATE_RATE_HZ"=4, "ACCEL_FSR_G"=5, "GYRO_FSR_DPS"=6, "OP_STATUS"=8, "CAL_STATUS"=9, "SELFTEST_STATUS"=10, "CAPABILITY_FLAGS_L"=11, "CAPABILITY_FLAGS_H"=12, "SENSOR_STATUS"=16, "TIMESTAMP"=18, "YAW"=22, "ROLL"=24, "PITCH"=26, "HEADING"=28, "FUSED_HEADING"=30, "ALTITUDE_I"=32, "ALTITUDE_D"=34, "LINERA_ACC_X"=36, "LINERA_ACC_Y"=38, "LINERA_ACC_Z"=40, "QUAT_W"=42, "QUAT_X"=44, "QUAT_Y"=46, "QUAT_Z"=48, "MPU_TEMP_C"=50, "GYRO_X"=52, "GYRO_Y"=54, "GYRO_Z"=56, "ACC_X"=58, "ACC_Y"=60, "ACC_Z"=62, "MAG_X"=64, "MAG_Y"=66, "MAG_Z"=68, "PRESSURE_I"=70, "PRESSURE_D"=72, "PRESSURE_TEMP"=74, "YAW_OFFSET"=76, "QUAT_OFFSET_W"=78, "QUAT_OFFSET_X"=80, "QUAT_OFFSET_Y"=82, "QUAT_OFFSET_Z"=84, "INTEGRATION_CONTROL"=86, "VELOCITY_X"=88, "VELOCITY_Y"=92, "VELOCITY_Z"=96, "DISPLACMENT_X"=100, "DISPLACMENT_Y"=104, "DISPLACEMENT_Z"=108] ("Device Register")
          w159 = T1 16 items=["WHOAMI"=0, "HW_REV"=1, "FW_VER_MAJOR"=2, "FW_VER_MINOR"=3, "UPDATE_RATE_HZ"=4, "ACCEL_FSR_G"=5, "GYRO_FSR_DPS"=6, "OP_STATUS"=8, "CAL_STATUS"=9, "SELFTEST_STATUS"=10, "CAPABILITY_FLAGS_L"=11, "CAPABILITY_FLAGS_H"=12, "SENSOR_STATUS"=16, "TIMESTAMP"=18, "YAW"=22, "ROLL"=24, "PITCH"=26, "HEADING"=28, "FUSED_HEADING"=30, "ALTITUDE_I"=32, "ALTITUDE_D"=34, "LINERA_ACC_X"=36, "LINERA_ACC_Y"=38, "LINERA_ACC_Z"=40, "QUAT_W"=42, "QUAT_X"=44, "QUAT_Y"=46, "QUAT_Z"=48, "MPU_TEMP_C"=50, "GYRO_X"=52, "GYRO_Y"=54, "GYRO_Z"=56, "ACC_X"=58, "ACC_Y"=60, "ACC_Z"=62, "MAG_X"=64, "MAG_Y"=66, "MAG_Z"=68, "PRESSURE_I"=70, "PRESSURE_D"=72, "PRESSURE_TEMP"=74, "YAW_OFFSET"=76, "QUAT_OFFSET_W"=78, "QUAT_OFFSET_X"=80, "QUAT_OFFSET_Y"=82, "QUAT_OFFSET_Z"=84, "INTEGRATION_CONTROL"=86, "VELOCITY_X"=88, "VELOCITY_Y"=92, "VELOCITY_Z"=96, "DISPLACMENT_X"=100, "DISPLACMENT_Y"=104, "DISPLACEMENT_Z"=108] ("Device Register")
          w165 = T1 8 items=["WHOAMI"=0, "HW_REV"=1, "FW_VER_MAJOR"=2, "FW_VER_MINOR"=3, "UPDATE_RATE_HZ"=4, "ACCEL_FSR_G"=5, "GYRO_FSR_DPS"=6, "OP_STATUS"=8, "CAL_STATUS"=9, "SELFTEST_STATUS"=10, "CAPABILITY_FLAGS_L"=11, "CAPABILITY_FLAGS_H"=12, "SENSOR_STATUS"=16, "TIMESTAMP"=18, "YAW"=22, "ROLL"=24, "PITCH"=26, "HEADING"=28, "FUSED_HEADING"=30, "ALTITUDE_I"=32, "ALTITUDE_D"=34, "LINERA_ACC_X"=36, "LINERA_ACC_Y"=38, "LINERA_ACC_Z"=40, "QUAT_W"=42, "QUAT_X"=44, "QUAT_Y"=46, "QUAT_Z"=48, "MPU_TEMP_C"=50, "GYRO_X"=52, "GYRO_Y"=54, "GYRO_Z"=56, "ACC_X"=58, "ACC_Y"=60, "ACC_Z"=62, "MAG_X"=64, "MAG_Y"=66, "MAG_Z"=68, "PRESSURE_I"=70, "PRESSURE_D"=72, "PRESSURE_TEMP"=74, "YAW_OFFSET"=76, "QUAT_OFFSET_W"=78, "QUAT_OFFSET_X"=80, "QUAT_OFFSET_Y"=82, "QUAT_OFFSET_Z"=84, "INTEGRATION_CONTROL"=86, "VELOCITY_X"=88, "VELOCITY_Y"=92, "VELOCITY_Z"=96, "DISPLACMENT_X"=100, "DISPLACMENT_Y"=104, "DISPLACEMENT_Z"=108] ("Device Register")
          n117 = in-place-match #19(w136) -> (w164:u8[])
          n118 = in-place-match #20(w135) -> (w162:u8[])
          n119 = Index Array(array=w162, index #1=54 ("index")) -> (element #1=w160:u8, element #2=w158:u8, element #3=w155:u8, element #4=w154:u8)  [unwired: 3 in]
          n120 = Replace Array Subset(array=w164, new element #1=w160, index #1=w165, new element #2=w158, index #2=w159, new element #3=w155, index #3=w157, new element #4=w154, index #4=w156) -> (w163:u8[])
          n121 = in-place-match #19(w163) -> (w134:u8[])
          n122 = in-place-match #20(w162) -> ()  [unwired: 1 out]
        }
      }
      frame "#p" {
        # "AHRSAndPositioning Update Packet"
        n123 = String Subset(string=w231, offset (0)=4) -> (substring=w233:string)  [unwired: 1 in]
        n124 = String To Byte Array(string=w233) -> (unsigned byte array=w232:u8[])
        n125 = in-place {
          w292 = T1 22 items=["WHOAMI"=0, "HW_REV"=1, "FW_VER_MAJOR"=2, "FW_VER_MINOR"=3, "UPDATE_RATE_HZ"=4, "ACCEL_FSR_G"=5, "GYRO_FSR_DPS"=6, "OP_STATUS"=8, "CAL_STATUS"=9, "SELFTEST_STATUS"=10, "CAPABILITY_FLAGS_L"=11, "CAPABILITY_FLAGS_H"=12, "SENSOR_STATUS"=16, "TIMESTAMP"=18, "YAW"=22, "ROLL"=24, "PITCH"=26, "HEADING"=28, "FUSED_HEADING"=30, "ALTITUDE_I"=32, "ALTITUDE_D"=34, "LINERA_ACC_X"=36, "LINERA_ACC_Y"=38, "LINERA_ACC_Z"=40, "QUAT_W"=42, "QUAT_X"=44, "QUAT_Y"=46, "QUAT_Z"=48, "MPU_TEMP_C"=50, "GYRO_X"=52, "GYRO_Y"=54, "GYRO_Z"=56, "ACC_X"=58, "ACC_Y"=60, "ACC_Z"=62, "MAG_X"=64, "MAG_Y"=66, "MAG_Z"=68, "PRESSURE_I"=70, "PRESSURE_D"=72, "PRESSURE_TEMP"=74, "YAW_OFFSET"=76, "QUAT_OFFSET_W"=78, "QUAT_OFFSET_X"=80, "QUAT_OFFSET_Y"=82, "QUAT_OFFSET_Z"=84, "INTEGRATION_CONTROL"=86, "VELOCITY_X"=88, "VELOCITY_Y"=92, "VELOCITY_Z"=96, "DISPLACMENT_X"=100, "DISPLACMENT_Y"=104, "DISPLACEMENT_Z"=108] ("Device Register")
          n126 = in-place-match #21(w230) -> (w291:u8[])
          n127 = in-place-match #22(w232) -> (w289:u8[])
          n128 = Array Subset(array=w289, index=0, length=8) -> (w293:u8[])
          n129 = Replace Array Subset(array=w291, new element=w293, index=w292) -> (w290:u8[])
          n130 = in-place-match #21(w290) -> (w229:u8[])
          n131 = in-place-match #22(w289) -> (w228:u8[])
        }
        n132 = in-place {
          w286 = T1 32 items=["WHOAMI"=0, "HW_REV"=1, "FW_VER_MAJOR"=2, "FW_VER_MINOR"=3, "UPDATE_RATE_HZ"=4, "ACCEL_FSR_G"=5, "GYRO_FSR_DPS"=6, "OP_STATUS"=8, "CAL_STATUS"=9, "SELFTEST_STATUS"=10, "CAPABILITY_FLAGS_L"=11, "CAPABILITY_FLAGS_H"=12, "SENSOR_STATUS"=16, "TIMESTAMP"=18, "YAW"=22, "ROLL"=24, "PITCH"=26, "HEADING"=28, "FUSED_HEADING"=30, "ALTITUDE_I"=32, "ALTITUDE_D"=34, "LINERA_ACC_X"=36, "LINERA_ACC_Y"=38, "LINERA_ACC_Z"=40, "QUAT_W"=42, "QUAT_X"=44, "QUAT_Y"=46, "QUAT_Z"=48, "MPU_TEMP_C"=50, "GYRO_X"=52, "GYRO_Y"=54, "GYRO_Z"=56, "ACC_X"=58, "ACC_Y"=60, "ACC_Z"=62, "MAG_X"=64, "MAG_Y"=66, "MAG_Z"=68, "PRESSURE_I"=70, "PRESSURE_D"=72, "PRESSURE_TEMP"=74, "YAW_OFFSET"=76, "QUAT_OFFSET_W"=78, "QUAT_OFFSET_X"=80, "QUAT_OFFSET_Y"=82, "QUAT_OFFSET_Z"=84, "INTEGRATION_CONTROL"=86, "VELOCITY_X"=88, "VELOCITY_Y"=92, "VELOCITY_Z"=96, "DISPLACMENT_X"=100, "DISPLACMENT_Y"=104, "DISPLACEMENT_Z"=108] ("Device Register")
          n133 = in-place-match #23(w229) -> (w285:u8[])
          n134 = in-place-match #24(w228) -> (w282:u8[])
          n135 = Array Subset(array=w282, index=8, length=4) -> (w283:u8[])
          n136 = Replace Array Subset(array=w285, new element=w283, index=w286) -> (w284:u8[])
          n137 = in-place-match #23(w284) -> (w227:u8[])
          n138 = in-place-match #24(w282) -> (w226:u8[])
        }
        n139 = in-place {
          w279 = T1 30 items=["WHOAMI"=0, "HW_REV"=1, "FW_VER_MAJOR"=2, "FW_VER_MINOR"=3, "UPDATE_RATE_HZ"=4, "ACCEL_FSR_G"=5, "GYRO_FSR_DPS"=6, "OP_STATUS"=8, "CAL_STATUS"=9, "SELFTEST_STATUS"=10, "CAPABILITY_FLAGS_L"=11, "CAPABILITY_FLAGS_H"=12, "SENSOR_STATUS"=16, "TIMESTAMP"=18, "YAW"=22, "ROLL"=24, "PITCH"=26, "HEADING"=28, "FUSED_HEADING"=30, "ALTITUDE_I"=32, "ALTITUDE_D"=34, "LINERA_ACC_X"=36, "LINERA_ACC_Y"=38, "LINERA_ACC_Z"=40, "QUAT_W"=42, "QUAT_X"=44, "QUAT_Y"=46, "QUAT_Z"=48, "MPU_TEMP_C"=50, "GYRO_X"=52, "GYRO_Y"=54, "GYRO_Z"=56, "ACC_X"=58, "ACC_Y"=60, "ACC_Z"=62, "MAG_X"=64, "MAG_Y"=66, "MAG_Z"=68, "PRESSURE_I"=70, "PRESSURE_D"=72, "PRESSURE_TEMP"=74, "YAW_OFFSET"=76, "QUAT_OFFSET_W"=78, "QUAT_OFFSET_X"=80, "QUAT_OFFSET_Y"=82, "QUAT_OFFSET_Z"=84, "INTEGRATION_CONTROL"=86, "VELOCITY_X"=88, "VELOCITY_Y"=92, "VELOCITY_Z"=96, "DISPLACMENT_X"=100, "DISPLACMENT_Y"=104, "DISPLACEMENT_Z"=108] ("Device Register")
          n140 = in-place-match #25(w227) -> (w278:u8[])
          n141 = in-place-match #26(w226) -> (w275:u8[])
          n142 = Array Subset(array=w275, index=12, length=2) -> (w276:u8[])
          n143 = Replace Array Subset(array=w278, new element=w276, index=w279) -> (w277:u8[])
          n144 = in-place-match #25(w277) -> (w225:u8[])
          n145 = in-place-match #26(w275) -> (w224:u8[])
        }
        n146 = in-place {
          w272 = T1 36 items=["WHOAMI"=0, "HW_REV"=1, "FW_VER_MAJOR"=2, "FW_VER_MINOR"=3, "UPDATE_RATE_HZ"=4, "ACCEL_FSR_G"=5, "GYRO_FSR_DPS"=6, "OP_STATUS"=8, "CAL_STATUS"=9, "SELFTEST_STATUS"=10, "CAPABILITY_FLAGS_L"=11, "CAPABILITY_FLAGS_H"=12, "SENSOR_STATUS"=16, "TIMESTAMP"=18, "YAW"=22, "ROLL"=24, "PITCH"=26, "HEADING"=28, "FUSED_HEADING"=30, "ALTITUDE_I"=32, "ALTITUDE_D"=34, "LINERA_ACC_X"=36, "LINERA_ACC_Y"=38, "LINERA_ACC_Z"=40, "QUAT_W"=42, "QUAT_X"=44, "QUAT_Y"=46, "QUAT_Z"=48, "MPU_TEMP_C"=50, "GYRO_X"=52, "GYRO_Y"=54, "GYRO_Z"=56, "ACC_X"=58, "ACC_Y"=60, "ACC_Z"=62, "MAG_X"=64, "MAG_Y"=66, "MAG_Z"=68, "PRESSURE_I"=70, "PRESSURE_D"=72, "PRESSURE_TEMP"=74, "YAW_OFFSET"=76, "QUAT_OFFSET_W"=78, "QUAT_OFFSET_X"=80, "QUAT_OFFSET_Y"=82, "QUAT_OFFSET_Z"=84, "INTEGRATION_CONTROL"=86, "VELOCITY_X"=88, "VELOCITY_Y"=92, "VELOCITY_Z"=96, "DISPLACMENT_X"=100, "DISPLACMENT_Y"=104, "DISPLACEMENT_Z"=108] ("Device Register")
          n147 = in-place-match #27(w225) -> (w271:u8[])
          n148 = in-place-match #28(w224) -> (w268:u8[])
          n149 = Array Subset(array=w268, index=14, length=6) -> (w269:u8[])
          n150 = Replace Array Subset(array=w271, new element=w269, index=w272) -> (w270:u8[])
          n151 = in-place-match #27(w270) -> (w223:u8[])
          n152 = in-place-match #28(w268) -> (w222:u8[])
        }
        n153 = in-place {
          w265 = T1 88 items=["WHOAMI"=0, "HW_REV"=1, "FW_VER_MAJOR"=2, "FW_VER_MINOR"=3, "UPDATE_RATE_HZ"=4, "ACCEL_FSR_G"=5, "GYRO_FSR_DPS"=6, "OP_STATUS"=8, "CAL_STATUS"=9, "SELFTEST_STATUS"=10, "CAPABILITY_FLAGS_L"=11, "CAPABILITY_FLAGS_H"=12, "SENSOR_STATUS"=16, "TIMESTAMP"=18, "YAW"=22, "ROLL"=24, "PITCH"=26, "HEADING"=28, "FUSED_HEADING"=30, "ALTITUDE_I"=32, "ALTITUDE_D"=34, "LINERA_ACC_X"=36, "LINERA_ACC_Y"=38, "LINERA_ACC_Z"=40, "QUAT_W"=42, "QUAT_X"=44, "QUAT_Y"=46, "QUAT_Z"=48, "MPU_TEMP_C"=50, "GYRO_X"=52, "GYRO_Y"=54, "GYRO_Z"=56, "ACC_X"=58, "ACC_Y"=60, "ACC_Z"=62, "MAG_X"=64, "MAG_Y"=66, "MAG_Z"=68, "PRESSURE_I"=70, "PRESSURE_D"=72, "PRESSURE_TEMP"=74, "YAW_OFFSET"=76, "QUAT_OFFSET_W"=78, "QUAT_OFFSET_X"=80, "QUAT_OFFSET_Y"=82, "QUAT_OFFSET_Z"=84, "INTEGRATION_CONTROL"=86, "VELOCITY_X"=88, "VELOCITY_Y"=92, "VELOCITY_Z"=96, "DISPLACMENT_X"=100, "DISPLACMENT_Y"=104, "DISPLACEMENT_Z"=108] ("Device Register")
          n154 = in-place-match #29(w223) -> (w264:u8[])
          n155 = in-place-match #30(w222) -> (w261:u8[])
          n156 = Array Subset(array=w261, index=20, length=24) -> (w262:u8[])
          n157 = Replace Array Subset(array=w264, new element=w262, index=w265) -> (w263:u8[])
          n158 = in-place-match #29(w263) -> (w221:u8[])
          n159 = in-place-match #30(w261) -> (w220:u8[])
        }
        n160 = in-place {
          w258 = T1 42 items=["WHOAMI"=0, "HW_REV"=1, "FW_VER_MAJOR"=2, "FW_VER_MINOR"=3, "UPDATE_RATE_HZ"=4, "ACCEL_FSR_G"=5, "GYRO_FSR_DPS"=6, "OP_STATUS"=8, "CAL_STATUS"=9, "SELFTEST_STATUS"=10, "CAPABILITY_FLAGS_L"=11, "CAPABILITY_FLAGS_H"=12, "SENSOR_STATUS"=16, "TIMESTAMP"=18, "YAW"=22, "ROLL"=24, "PITCH"=26, "HEADING"=28, "FUSED_HEADING"=30, "ALTITUDE_I"=32, "ALTITUDE_D"=34, "LINERA_ACC_X"=36, "LINERA_ACC_Y"=38, "LINERA_ACC_Z"=40, "QUAT_W"=42, "QUAT_X"=44, "QUAT_Y"=46, "QUAT_Z"=48, "MPU_TEMP_C"=50, "GYRO_X"=52, "GYRO_Y"=54, "GYRO_Z"=56, "ACC_X"=58, "ACC_Y"=60, "ACC_Z"=62, "MAG_X"=64, "MAG_Y"=66, "MAG_Z"=68, "PRESSURE_I"=70, "PRESSURE_D"=72, "PRESSURE_TEMP"=74, "YAW_OFFSET"=76, "QUAT_OFFSET_W"=78, "QUAT_OFFSET_X"=80, "QUAT_OFFSET_Y"=82, "QUAT_OFFSET_Z"=84, "INTEGRATION_CONTROL"=86, "VELOCITY_X"=88, "VELOCITY_Y"=92, "VELOCITY_Z"=96, "DISPLACMENT_X"=100, "DISPLACMENT_Y"=104, "DISPLACEMENT_Z"=108] ("Device Register")
          n161 = in-place-match #31(w221) -> (w257:u8[])
          n162 = in-place-match #32(w220) -> (w254:u8[])
          n163 = Array Subset(array=w254, index=44, length=8) -> (w255:u8[])
          n164 = Replace Array Subset(array=w257, new element=w255, index=w258) -> (w256:u8[])
          n165 = in-place-match #31(w256) -> (w219:u8[])
          n166 = in-place-match #32(w254) -> (w218:u8[])
        }
        n167 = in-place {
          w251 = T1 50 items=["WHOAMI"=0, "HW_REV"=1, "FW_VER_MAJOR"=2, "FW_VER_MINOR"=3, "UPDATE_RATE_HZ"=4, "ACCEL_FSR_G"=5, "GYRO_FSR_DPS"=6, "OP_STATUS"=8, "CAL_STATUS"=9, "SELFTEST_STATUS"=10, "CAPABILITY_FLAGS_L"=11, "CAPABILITY_FLAGS_H"=12, "SENSOR_STATUS"=16, "TIMESTAMP"=18, "YAW"=22, "ROLL"=24, "PITCH"=26, "HEADING"=28, "FUSED_HEADING"=30, "ALTITUDE_I"=32, "ALTITUDE_D"=34, "LINERA_ACC_X"=36, "LINERA_ACC_Y"=38, "LINERA_ACC_Z"=40, "QUAT_W"=42, "QUAT_X"=44, "QUAT_Y"=46, "QUAT_Z"=48, "MPU_TEMP_C"=50, "GYRO_X"=52, "GYRO_Y"=54, "GYRO_Z"=56, "ACC_X"=58, "ACC_Y"=60, "ACC_Z"=62, "MAG_X"=64, "MAG_Y"=66, "MAG_Z"=68, "PRESSURE_I"=70, "PRESSURE_D"=72, "PRESSURE_TEMP"=74, "YAW_OFFSET"=76, "QUAT_OFFSET_W"=78, "QUAT_OFFSET_X"=80, "QUAT_OFFSET_Y"=82, "QUAT_OFFSET_Z"=84, "INTEGRATION_CONTROL"=86, "VELOCITY_X"=88, "VELOCITY_Y"=92, "VELOCITY_Z"=96, "DISPLACMENT_X"=100, "DISPLACMENT_Y"=104, "DISPLACEMENT_Z"=108] ("Device Register")
          n168 = in-place-match #33(w219) -> (w250:u8[])
          n169 = in-place-match #34(w218) -> (w247:u8[])
          n170 = Array Subset(array=w247, index=52, length=2) -> (w248:u8[])
          n171 = Replace Array Subset(array=w250, new element=w248, index=w251) -> (w249:u8[])
          n172 = in-place-match #33(w249) -> (w217:u8[])
          n173 = in-place-match #34(w247) -> (w216:u8[])
        }
        n174 = in-place {
          w237 = T1 10 items=["WHOAMI"=0, "HW_REV"=1, "FW_VER_MAJOR"=2, "FW_VER_MINOR"=3, "UPDATE_RATE_HZ"=4, "ACCEL_FSR_G"=5, "GYRO_FSR_DPS"=6, "OP_STATUS"=8, "CAL_STATUS"=9, "SELFTEST_STATUS"=10, "CAPABILITY_FLAGS_L"=11, "CAPABILITY_FLAGS_H"=12, "SENSOR_STATUS"=16, "TIMESTAMP"=18, "YAW"=22, "ROLL"=24, "PITCH"=26, "HEADING"=28, "FUSED_HEADING"=30, "ALTITUDE_I"=32, "ALTITUDE_D"=34, "LINERA_ACC_X"=36, "LINERA_ACC_Y"=38, "LINERA_ACC_Z"=40, "QUAT_W"=42, "QUAT_X"=44, "QUAT_Y"=46, "QUAT_Z"=48, "MPU_TEMP_C"=50, "GYRO_X"=52, "GYRO_Y"=54, "GYRO_Z"=56, "ACC_X"=58, "ACC_Y"=60, "ACC_Z"=62, "MAG_X"=64, "MAG_Y"=66, "MAG_Z"=68, "PRESSURE_I"=70, "PRESSURE_D"=72, "PRESSURE_TEMP"=74, "YAW_OFFSET"=76, "QUAT_OFFSET_W"=78, "QUAT_OFFSET_X"=80, "QUAT_OFFSET_Y"=82, "QUAT_OFFSET_Z"=84, "INTEGRATION_CONTROL"=86, "VELOCITY_X"=88, "VELOCITY_Y"=92, "VELOCITY_Z"=96, "DISPLACMENT_X"=100, "DISPLACMENT_Y"=104, "DISPLACEMENT_Z"=108] ("Device Register")
          w238 = T1 9 items=["WHOAMI"=0, "HW_REV"=1, "FW_VER_MAJOR"=2, "FW_VER_MINOR"=3, "UPDATE_RATE_HZ"=4, "ACCEL_FSR_G"=5, "GYRO_FSR_DPS"=6, "OP_STATUS"=8, "CAL_STATUS"=9, "SELFTEST_STATUS"=10, "CAPABILITY_FLAGS_L"=11, "CAPABILITY_FLAGS_H"=12, "SENSOR_STATUS"=16, "TIMESTAMP"=18, "YAW"=22, "ROLL"=24, "PITCH"=26, "HEADING"=28, "FUSED_HEADING"=30, "ALTITUDE_I"=32, "ALTITUDE_D"=34, "LINERA_ACC_X"=36, "LINERA_ACC_Y"=38, "LINERA_ACC_Z"=40, "QUAT_W"=42, "QUAT_X"=44, "QUAT_Y"=46, "QUAT_Z"=48, "MPU_TEMP_C"=50, "GYRO_X"=52, "GYRO_Y"=54, "GYRO_Z"=56, "ACC_X"=58, "ACC_Y"=60, "ACC_Z"=62, "MAG_X"=64, "MAG_Y"=66, "MAG_Z"=68, "PRESSURE_I"=70, "PRESSURE_D"=72, "PRESSURE_TEMP"=74, "YAW_OFFSET"=76, "QUAT_OFFSET_W"=78, "QUAT_OFFSET_X"=80, "QUAT_OFFSET_Y"=82, "QUAT_OFFSET_Z"=84, "INTEGRATION_CONTROL"=86, "VELOCITY_X"=88, "VELOCITY_Y"=92, "VELOCITY_Z"=96, "DISPLACMENT_X"=100, "DISPLACMENT_Y"=104, "DISPLACEMENT_Z"=108] ("Device Register")
          w240 = T1 16 items=["WHOAMI"=0, "HW_REV"=1, "FW_VER_MAJOR"=2, "FW_VER_MINOR"=3, "UPDATE_RATE_HZ"=4, "ACCEL_FSR_G"=5, "GYRO_FSR_DPS"=6, "OP_STATUS"=8, "CAL_STATUS"=9, "SELFTEST_STATUS"=10, "CAPABILITY_FLAGS_L"=11, "CAPABILITY_FLAGS_H"=12, "SENSOR_STATUS"=16, "TIMESTAMP"=18, "YAW"=22, "ROLL"=24, "PITCH"=26, "HEADING"=28, "FUSED_HEADING"=30, "ALTITUDE_I"=32, "ALTITUDE_D"=34, "LINERA_ACC_X"=36, "LINERA_ACC_Y"=38, "LINERA_ACC_Z"=40, "QUAT_W"=42, "QUAT_X"=44, "QUAT_Y"=46, "QUAT_Z"=48, "MPU_TEMP_C"=50, "GYRO_X"=52, "GYRO_Y"=54, "GYRO_Z"=56, "ACC_X"=58, "ACC_Y"=60, "ACC_Z"=62, "MAG_X"=64, "MAG_Y"=66, "MAG_Z"=68, "PRESSURE_I"=70, "PRESSURE_D"=72, "PRESSURE_TEMP"=74, "YAW_OFFSET"=76, "QUAT_OFFSET_W"=78, "QUAT_OFFSET_X"=80, "QUAT_OFFSET_Y"=82, "QUAT_OFFSET_Z"=84, "INTEGRATION_CONTROL"=86, "VELOCITY_X"=88, "VELOCITY_Y"=92, "VELOCITY_Z"=96, "DISPLACMENT_X"=100, "DISPLACMENT_Y"=104, "DISPLACEMENT_Z"=108] ("Device Register")
          w246 = T1 8 items=["WHOAMI"=0, "HW_REV"=1, "FW_VER_MAJOR"=2, "FW_VER_MINOR"=3, "UPDATE_RATE_HZ"=4, "ACCEL_FSR_G"=5, "GYRO_FSR_DPS"=6, "OP_STATUS"=8, "CAL_STATUS"=9, "SELFTEST_STATUS"=10, "CAPABILITY_FLAGS_L"=11, "CAPABILITY_FLAGS_H"=12, "SENSOR_STATUS"=16, "TIMESTAMP"=18, "YAW"=22, "ROLL"=24, "PITCH"=26, "HEADING"=28, "FUSED_HEADING"=30, "ALTITUDE_I"=32, "ALTITUDE_D"=34, "LINERA_ACC_X"=36, "LINERA_ACC_Y"=38, "LINERA_ACC_Z"=40, "QUAT_W"=42, "QUAT_X"=44, "QUAT_Y"=46, "QUAT_Z"=48, "MPU_TEMP_C"=50, "GYRO_X"=52, "GYRO_Y"=54, "GYRO_Z"=56, "ACC_X"=58, "ACC_Y"=60, "ACC_Z"=62, "MAG_X"=64, "MAG_Y"=66, "MAG_Z"=68, "PRESSURE_I"=70, "PRESSURE_D"=72, "PRESSURE_TEMP"=74, "YAW_OFFSET"=76, "QUAT_OFFSET_W"=78, "QUAT_OFFSET_X"=80, "QUAT_OFFSET_Y"=82, "QUAT_OFFSET_Z"=84, "INTEGRATION_CONTROL"=86, "VELOCITY_X"=88, "VELOCITY_Y"=92, "VELOCITY_Z"=96, "DISPLACMENT_X"=100, "DISPLACMENT_Y"=104, "DISPLACEMENT_Z"=108] ("Device Register")
          n175 = in-place-match #35(w217) -> (w245:u8[])
          n176 = in-place-match #36(w216) -> (w243:u8[])
          n177 = Index Array(array=w243, index #1=54 ("index")) -> (element #1=w241:u8, element #2=w239:u8, element #3=w236:u8, element #4=w235:u8)  [unwired: 3 in]
          n178 = Replace Array Subset(array=w245, new element #1=w241, index #1=w246, new element #2=w239, index #2=w240, new element #3=w236, index #3=w238, new element #4=w235, index #4=w237) -> (w244:u8[])
          n179 = in-place-match #35(w244) -> (w215:u8[])
          n180 = in-place-match #36(w243) -> ()  [unwired: 1 out]
        }
      }
      frame "#i" {
        # "Board Identity Response Packet"
        n181 = String Subset(string=w299, offset (0)=4) -> (substring=w300:string)  [unwired: 1 in]
        n182 = String To Byte Array(string=w300) -> (unsigned byte array=w298:u8[])
        n183 = in-place {
          w306 = T1 0 items=["WHOAMI"=0, "HW_REV"=1, "FW_VER_MAJOR"=2, "FW_VER_MINOR"=3, "UPDATE_RATE_HZ"=4, "ACCEL_FSR_G"=5, "GYRO_FSR_DPS"=6, "OP_STATUS"=8, "CAL_STATUS"=9, "SELFTEST_STATUS"=10, "CAPABILITY_FLAGS_L"=11, "CAPABILITY_FLAGS_H"=12, "SENSOR_STATUS"=16, "TIMESTAMP"=18, "YAW"=22, "ROLL"=24, "PITCH"=26, "HEADING"=28, "FUSED_HEADING"=30, "ALTITUDE_I"=32, "ALTITUDE_D"=34, "LINERA_ACC_X"=36, "LINERA_ACC_Y"=38, "LINERA_ACC_Z"=40, "QUAT_W"=42, "QUAT_X"=44, "QUAT_Y"=46, "QUAT_Z"=48, "MPU_TEMP_C"=50, "GYRO_X"=52, "GYRO_Y"=54, "GYRO_Z"=56, "ACC_X"=58, "ACC_Y"=60, "ACC_Z"=62, "MAG_X"=64, "MAG_Y"=66, "MAG_Z"=68, "PRESSURE_I"=70, "PRESSURE_D"=72, "PRESSURE_TEMP"=74, "YAW_OFFSET"=76, "QUAT_OFFSET_W"=78, "QUAT_OFFSET_X"=80, "QUAT_OFFSET_Y"=82, "QUAT_OFFSET_Z"=84, "INTEGRATION_CONTROL"=86, "VELOCITY_X"=88, "VELOCITY_Y"=92, "VELOCITY_Z"=96, "DISPLACMENT_X"=100, "DISPLACMENT_Y"=104, "DISPLACEMENT_Z"=108] ("Device Register")
          n184 = in-place-match #37(w297) -> (w305:u8[])
          n185 = in-place-match #38(w298) -> (w302:u8[])
          n186 = Array Subset(array=w302, index=0, length=4) -> (w303:u8[])
          n187 = Replace Array Subset(array=w305, new element=w303, index=w306) -> (w304:u8[])
          n188 = in-place-match #37(w304) -> (w296:u8[])
          n189 = in-place-match #38(w302) -> ()  [unwired: 1 out]
        }
      }
    }
    n190 = in-place-match #2(w24) -> (→"Data":u8[])
  }
  "Packet" <- "Packet"
  "error out" <- "error in (no error)"
